vi "Pull Behavior_MWMATHIS.vi"(7 "Water Reward File":path=path "C:/Users/Mackenzie Amoroso/Desktop/REWARD_ente7102015") -> ()   [LabVIEW 2012] (continued)
, "mag"=0.0, "move time"=400.0, "timeout"=1000.0, "watertime"=100.0, "magtime"=25.0, "light"=0.0}, {"home Y2"=3.0, "home X2"=2.8, "home Y1"=2.0, "home X1"=2.4, "home TO"=500.0, "start Y2"=2.7, "start X2"=2.35, "start Y1 "=2.0, "start X1"=2.0, "start TO"=0.0, "end Y2"=2.6, "end X2"=2.2, "end Y1"=2.5, "end X1"=1.8, "end TO"=50.0, "mag"=0.0, "move time"=400.0, "timeout"=1000.0, "watertime"=100.0, "magtime"=25.0, "light"=0.0}, {"home Y2"=3.0, "home X2"=2.8, "home Y1"=2.0, "home X1"=2.4, "home TO"=500.0, "start Y2"=2.7, "start X2"=2.35, "start Y1 "=2.0, "start X1"=2.0, "start TO"=0.0, "end Y2"=2.6, "end X2"=2.2, "end Y1"=2.5, "end X1"=1.8, "end TO"=50.0, "mag"=0.0, "move time"=400.0, "timeout"=1000.0, "watertime"=100.0, "magtime"=25.0, "light"=0.0}, {"home Y2"=3.0, "home X2"=2.8, "home Y1"=2.0, "home X1"=2.4, "home TO"=500.0, "start Y2"=2.7, "start X2"=2.35, "start Y1 "=2.0, "start X1"=2.0, "start TO"=0.0, "end Y2"=2.6, "end X2"=2.2, "end Y1"=2.5, "end X1"=1.8, "end TO"=50.0, "mag"=0.0, "move time"=400.0, "timeout"=1000.0, "watertime"=100.0, "magtime"=25.0, "light"=0.0}, {"home Y2"=3.0, "home X2"=2.8, "home Y1"=2.0, "home X1"=2.4, "home TO"=500.0, "start Y2"=2.7, "start X2"=2.35, "start Y1 "=2.0, "start X1"=2.0, "start TO"=0.0, "end Y2"=2.6, "end X2"=2.2, "end Y1"=2.5, "end X1"=1.8, "end TO"=50.0, "mag"=0.0, "move time"=400.0, "timeout"=1000.0, "watertime"=100.0, "magtime"=25.0, "light"=0.0}, {"home Y2"=3.0, "home X2"=2.8, "home Y1"=2.0, "home X1"=2.4, "home TO"=500.0, "start Y2"=2.7, "start X2"=2.35, "start Y1 "=2.0, "start X1"=2.0, "start TO"=0.0, "end Y2"=2.6, "end X2"=2.2, "end Y1"=2.5, "end X1"=1.8, "end TO"=50.0, "mag"=0.0, "move time"=400.0, "timeout"=1000.0, "watertime"=100.0, "magtime"=25.0, "light"=0.0}, {"home Y2"=3.0, "home X2"=2.8, "home Y1"=2.0, "home X1"=2.4, "home TO"=500.0, "start Y2"=2.7, "start X2"=2.35, "start Y1 "=2.0, "start X1"=2.0, "start TO"=0.0, "end Y2"=2.6, "end X2"=2.2, "end Y1"=2.5, "end X1"=1.8, "end TO"=50.0, "mag"=0.0, "move time"=400.0, "timeout"=1000.0, "watertime"=100.0, "magtime"=25.0, "light"=0.0}, {"home Y2"=3.0, "home X2"=2.8, "home Y1"=2.0, "home X1"=2.4, "home TO"=500.0, "start Y2"=2.7, "start X2"=2.35, "start Y1 "=2.0, "start X1"=2.0, "start TO"=0.0, "end Y2"=2.6, "end X2"=2.2, "end Y1"=2.5, "end X1"=1.8, "end TO"=50.0, "mag"=0.0, "move time"=400.0, "timeout"=1000.0, "watertime"=100.0, "magtime"=25.0, "light"=0.0}, {"home Y2"=3.0, "home X2"=2.8, "home Y1"=2.0, "home X1"=2.4, "home TO"=500.0, "start Y2"=2.7, "start X2"=2.35, "start Y1 "=2.0, "start X1"=2.0, "start TO"=0.0, "end Y2"=2.6, "end X2"=2.2, "end Y1"=2.5, "end X1"=1.8, "end TO"=50.0, "mag"=0.0, "move time"=400.0, "timeout"=1000.0, "watertime"=100.0, "magtime"=25.0, "light"=0.0}, {"home Y2"=3.0, "home X2"=2.8, "home Y1"=2.0, "home X1"=2.4, "home TO"=500.0, "start Y2"=2.7, "start X2"=2.35, "start Y1 "=2.0, "start X1"=2.0, "start TO"=0.0, "end Y2"=2.6, "end X2"=2.2, "end Y1"=2.5, "end X1"=1.8, "end TO"=50.0, "mag"=0.0, "move time"=400.0, "timeout"=1000.0, "watertime"=100.0, "magtime"=25.0, "light"=0.0}, {"home Y2"=3.0, "home X2"=2.8, "home Y1"=2.0, "home X1"=2.4, "home TO"=500.0, "start Y2"=2.7, "start X2"=2.35, "start Y1 "=2.0, "start X1"=2.0, "start TO"=0.0, "end Y2"=2.6, "end X2"=2.2, "end Y1"=2.5, "end X1"=1.8, "end TO"=50.0, "mag"=0.0, "move time"=400.0, "timeout"=1000.0, "watertime"=100.0, "magtime"=25.0, "light"=0.0}, {"home Y2"=3.0, "home X2"=2.8, "home Y1"=2.0, "home X1"=2.4, "home TO"=500.0, "start Y2"=2.7, "start X2"=2.35, "start Y1 "=2.0, "start X1"=2.0, "start TO"=0.0, "end Y2"=2.6, "end X2"=2.2, "end Y1"=2.5, "end X1"=1.8, "end TO"=50.0, "mag"=0.0, "move time"=400.0, "timeout"=1000.0, "watertime"=100.0, "magtime"=25.0, "light"=0.0}, {"home Y2"=3.0, "home X2"=2.8, "home Y1"=2.0, "home X1"=2.4, "home TO"=500.0, "start Y2"=2.7, "start X2"=2.35, "start Y1 "=2.0, "start X1"=2.0, "start TO"=0.0, "end Y2"=2.6, "end X2"=2.2, "end Y1"=2.5, "end X1"=1.8, "end TO"=50.0, "mag"=0.0, "move time"=400.0, "timeout"=1000.0, "watertime"=100.0, "magtime"=25.0, "light"=0.0}, {"home Y2"=3.0, "home X2"=2.8, "home Y1"=2.0, "home X1"=2.4, "home TO"=500.0, "start Y2"=2.7, "start X2"=2.35, "start Y1 "=2.0, "start X1"=2.0, "start TO"=0.0, "end Y2"=2.6, "end X2"=2.2, "end Y1"=2.5, "end X1"=1.8, "end TO"=50.0, "mag"=0.0, "move time"=400.0, "timeout"=1000.0, "watertime"=100.0, "magtime"=25.0, "light"=0.0}, {"home Y2"=3.0, "home X2"=2.8, "home Y1"=2.0, "home X1"=2.4, "home TO"=500.0, "start Y2"=2.7, "start X2"=2.35, "start Y1 "=2.0, "start X1"=2.0, "start TO"=0.0, "end Y2"=2.6, "end X2"=2.2, "end Y1"=2.5, "end X1"=1.8, "end TO"=50.0, "mag"=0.0, "move time"=400.0, "timeout"=1000.0, "watertime"=100.0, "magtime"=25.0, "light"=0.0}, {"home Y2"=3.0, "home X2"=2.8, "home Y1"=2.0, "home X1"=2.4, "home TO"=500.0, "start Y2"=2.7, "start X2"=2.35, "start Y1 "=2.0, "start X1"=2.0, "start TO"=0.0, "end Y2"=2.6, "end X2"=2.2, "end Y1"=2.5, "end X1"=1.8, "end TO"=50.0, "mag"=0.0, "move time"=400.0, "timeout"=1000.0, "watertime"=100.0, "magtime"=25.0, "light"=0.0}, {"home Y2"=3.0, "home X2"=2.8, "home Y1"=2.0, "home X1"=2.4, "home TO"=500.0, "start Y2"=2.7, "start X2"=2.35, "start Y1 "=2.0, "start X1"=2.0, "start TO"=0.0, "end Y2"=2.6, "end X2"=2.2, "end Y1"=2.5, "end X1"=1.8, "end TO"=50.0, "mag"=0.0, "move time"=400.0, "timeout"=1000.0, "watertime"=100.0, "magtime"=25.0, "light"=0.0}, {"home Y2"=3.0, "home X2"=2.8, "home Y1"=2.0, "home X1"=2.4, "home TO"=500.0, "start Y2"=2.7, "start X2"=2.35, "start Y1 "=2.0, "start X1"=2.0, "start TO"=0.0, "end Y2"=2.6, "end X2"=2.2, "end Y1"=2.5, "end X1"=1.8, "end TO"=50.0, "mag"=0.0, "move time"=400.0, "timeout"=1000.0, "watertime"=100.0, "magtime"=25.0, "light"=0.0}, {"home Y2"=3.0, "home X2"=2.8, "home Y1"=2.0, "home X1"=2.4, "home TO"=500.0, "start Y2"=2.7, "start X2"=2.35, "start Y1 "=2.0, "start X1"=2.0, "start TO"=0.0, "end Y2"=2.6, "end X2"=2.2, "end Y1"=2.5, "end X1"=1.8, "end TO"=50.0, "mag"=0.0, "move time"=400.0, "timeout"=1000.0, "watertime"=100.0, "magtime"=25.0, "light"=0.0}, {"home Y2"=3.0, "home X2"=2.8, "home Y1"=2.0, "home X1"=2.4, "home TO"=500.0, "start Y2"=2.7, "start X2"=2.35, "start Y1 "=2.0, "start X1"=2.0, "start TO"=0.0, "end Y2"=2.6, "end X2"=2.2, "end Y1"=2.5, "end X1"=1.8, "end TO"=50.0, "mag"=0.0, "move time"=400.0, "timeout"=1000.0, "watertime"=100.0, "magtime"=25.0, "light"=0.0}, {"home Y2"=3.0, "home X2"=2.8, "home Y1"=2.0, "home X1"=2.4, "home TO"=500.0, "start Y2"=2.7, "start X2"=2.35, "start Y1 "=2.0, "start X1"=2.0, "start TO"=0.0, "end Y2"=2.6, "end X2"=2.2, "end Y1"=2.5, "end X1"=1.8, "end TO"=50.0, "mag"=0.0, "move time"=400.0, "timeout"=1000.0, "watertime"=100.0, "magtime"=25.0, "light"=0.0}, {"home Y2"=3.0, "home X2"=2.8, "home Y1"=2.0, "home X1"=2.4, "home TO"=500.0, "start Y2"=2.7, "start X2"=2.35, "start Y1 "=2.0, "start X1"=2.0, "start TO"=0.0, "end Y2"=2.6, "end X2"=2.2, "end Y1"=2.5, "end X1"=1.8, "end TO"=50.0, "mag"=0.0, "move time"=400.0, "timeout"=1000.0, "watertime"=100.0, "magtime"=25.0, "light"=0.0}, {"home Y2"=3.0, "home X2"=2.8, "home Y1"=2.0, "home X1"=2.4, "home TO"=500.0, "start Y2"=2.7, "start X2"=2.35, "start Y1 "=2.0, "start X1"=2.0, "start TO"=0.0, "end Y2"=2.6, "end X2"=2.2, "end Y1"=2.5, "end X1"=1.8, "end TO"=50.0, "mag"=0.0, "move time"=400.0, "timeout"=1000.0, "watertime"=100.0, "magtime"=25.0, "light"=0.0}, {"home Y2"=3.0, "home X2"=2.8, "home Y1"=2.0, "home X1"=2.4, "home TO"=500.0, "start Y2"=2.7, "start X2"=2.35, "start Y1 "=2.0, "start X1"=2.0, "start TO"=0.0, "end Y2"=2.6, "end X2"=2.2, "end Y1"=2.5, "end X1"=1.8, "end TO"=50.0, "mag"=0.0, "move time"=400.0, "timeout"=1000.0, "watertime"=100.0, "magtime"=25.0, "light"=0.0}, {"home Y2"=3.0, "home X2"=2.8, "home Y1"=2.0, "home X1"=2.4, "home TO"=500.0, "start Y2"=2.7, "start X2"=2.35, "start Y1 "=2.0, "start X1"=2.0, "start TO"=0.0, "end Y2"=2.6, "end X2"=2.2, "end Y1"=2.5, "end X1"=1.8, "end TO"=50.0, "mag"=0.0, "move time"=400.0, "timeout"=1000.0, "watertime"=100.0, "magtime"=25.0, "light"=0.0}, {"home Y2"=3.0, "home X2"=2.8, "home Y1"=2.0, "home X1"=2.4, "home TO"=500.0, "start Y2"=2.7, "start X2"=2.35, "start Y1 "=2.0, "start X1"=2.0, "start TO"=0.0, "end Y2"=2.6, "end X2"=2.2, "end Y1"=2.5, "end X1"=1.8, "end TO"=50.0, "mag"=0.0, "move time"=400.0, "timeout"=1000.0, "watertime"=100.0, "magtime"=25.0, "light"=0.0}, {"home Y2"=3.0, "home X2"=2.8, "home Y1"=2.0, "home X1"=2.4, "home TO"=500.0, "start Y2"=2.7, "start X2"=2.35, "start Y1 "=2.0, "start X1"=2.0, "start TO"=0.0, "end Y2"=2.6, "end X2"=2.2, "end Y1"=2.5, "end X1"=1.8, "end TO"=50.0, "mag"=0.0, "move time"=400.0, "timeout"=1000.0, "watertime"=100.0, "magtime"=25.0, "light"=0.0}, {"home Y2"=3.0, "home X2"=2.8, "home Y1"=2.0, "home X1"=2.4, "home TO"=500.0, "start Y2"=2.7, "start X2"=2.35, "start Y1 "=2.0, "start X1"=2.0, "start TO"=0.0, "end Y2"=2.6, "end X2"=2.2, "end Y1"=2.5, "end X1"=1.8, "end TO"=50.0, "mag"=0.0, "move time"=400.0, "timeout"=1000.0, "watertime"=100.0, "magtime"=25.0, "light"=0.0}, {"home Y2"=3.0, "home X2"=2.8, "home Y1"=2.0, "home X1"=2.4, "home TO"=500.0, "start Y2"=2.7, "start X2"=2.35, "start Y1 "=2.0, "start X1"=2.0, "start TO"=0.0, "end Y2"=2.6, "end X2"=2.2, "end Y1"=2.5, "end X1"=1.8, "end TO"=50.0, "mag"=0.0, "move time"=400.0, "timeout"=1000.0, "watertime"=100.0, "magtime"=25.0, "light"=0.0}, {"home Y2"=3.0, "home X2"=2.8, "home Y1"=2.0, "home X1"=2.4, "home TO"=500.0, "start Y2"=2.7, "start X2"=2.35, "start Y1 "=2.0, "start X1"=2.0, "start TO"=0.0, "end Y2"=2.6, "end X2"=2.2, "end Y1"=2.5, "end X1"=1.8, "end TO"=50.0, "mag"=0.0, "move time"=400.0, "timeout"=1000.0, "watertime"=100.0, "magtime"=25.0, "light"=0.0}, {"home Y2"=3.0, "home X2"=2.8, "home Y1"=2.0, "home X1"=2.4, "home TO"=500.0, "start Y2"=2.7, "start X2"=2.35, "start Y1 "=2.0, "start X1"=2.0, "start TO"=0.0, "end Y2"=2.6, "end X2"=2.2, "end Y1"=2.5, "end X1"=1.8, "end TO"=50.0, "mag"=0.0, "move time"=400.0, "timeout"=1000.0, "watertime"=100.0, "magtime"=25.0, "light"=0.0}, {"home Y2"=3.0, "home X2"=2.8, "home Y1"=2.0, "home X1"=2.4, "home TO"=500.0, "start Y2"=2.7, "start X2"=2.35, "start Y1 "=2.0, "start X1"=2.0, "start TO"=0.0, "end Y2"=2.6, "end X2"=2.2, "end Y1"=2.5, "end X1"=1.8, "end TO"=50.0, "mag"=0.0, "move time"=400.0, "timeout"=1000.0, "watertime"=100.0, "magtime"=25.0, "light"=0.0}, {"home Y2"=3.0, "home X2"=2.8, "home Y1"=2.0, "home X1"=2.4, "home TO"=500.0, "start Y2"=2.7, "start X2"=2.35, "start Y1 "=2.0, "start X1"=2.0, "start TO"=0.0, "end Y2"=2.6, "end X2"=2.2, "end Y1"=2.5, "end X1"=1.8, "end TO"=50.0, "mag"=0.0, "move time"=400.0, "timeout"=1000.0, "watertime"=100.0, "magtime"=25.0, "light"=0.0}, {"home Y2"=3.0, "home X2"=2.8, "home Y1"=2.0, "home X1"=2.4, "home TO"=500.0, "start Y2"=2.7, "start X2"=2.35, "start Y1 "=2.0, "start X1"=2.0, "start TO"=0.0, "end Y2"=2.6, "end X2"=2.2, "end Y1"=2.5, "end X1"=1.8, "end TO"=50.0, "mag"=0.0, "move time"=400.0, "timeout"=1000.0, "watertime"=100.0, "magtime"=25.0, "light"=0.0}, {"home Y2"=3.0, "home X2"=2.8, "home Y1"=2.0, "home X1"=2.4, "home TO"=500.0, "start Y2"=2.7, "start X2"=2.35, "start Y1 "=2.0, "start X1"=2.0, "start TO"=0.0, "end Y2"=2.6, "end X2"=2.2, "end Y1"=2.5, "end X1"=1.8, "end TO"=50.0, "mag"=0.0, "move time"=400.0, "timeout"=1000.0, "watertime"=100.0, "magtime"=25.0, "light"=0.0}, {"home Y2"=3.0, "home X2"=2.8, "home Y1"=2.0, "home X1"=2.4, "home TO"=500.0, "start Y2"=2.7, "start X2"=2.35, "start Y1 "=2.0, "start X1"=2.0, "start TO"=0.0, "end Y2"=2.6, "end X2"=2.2, "end Y1"=2.5, "end X1"=1.8, "end TO"=50.0, "mag"=0.0, "move time"=400.0, "timeout"=1000.0, "watertime"=100.0, "magtime"=25.0, "light"=0.0}, {"home Y2"=3.0, "home X2"=2.8, "home Y1"=2.0, "home X1"=2.4, "home TO"=500.0, "start Y2"=2.7, "start X2"=2.35, "start Y1 "=2.0, "start X1"=2.0, "start TO"=0.0, "end Y2"=2.6, "end X2"=2.2, "end Y1"=2.5, "end X1"=1.8, "end TO"=50.0, "mag"=0.0, "move time"=400.0, "timeout"=1000.0, "watertime"=100.0, "magtime"=25.0, "light"=0.0}, {"home Y2"=3.0, "home X2"=2.8, "home Y1"=2.0, "home X1"=2.4, "home TO"=500.0, "start Y2"=2.7, "start X2"=2.35, "start Y1 "=2.0, "start X1"=2.0, "start TO"=0.0, "end Y2"=2.6, "end X2"=2.2, "end Y1"=2.5, "end X1"=1.8, "end TO"=50.0, "mag"=0.0, "move time"=400.0, "timeout"=1000.0, "watertime"=100.0, "magtime"=25.0, "light"=0.0}, {"home Y2"=0.0, "home X2"=0.0, "home Y1"=0.0, "home X1"=0.0, "home TO"=0.0, "start Y2"=0.0, "start X2"=0.0, "start Y1 "=0.0, "start X1"=0.0, "start TO"=0.0, "end Y2"=0.0, "end X2"=0.0, "end Y1"=0.0, "end X1"=0.0, "end TO"=0.0, "mag"=0.0, "move time"=0.0, "timeout"=0.0, "watertime"=0.0, "magtime"=0.0, "light"=0.0}, {"home Y2"=0.0, "home X2"=0.0, "home Y1"=0.0, "home X1"=0.0, "home TO"=0.0, "start Y2"=0.0, "start X2"=0.0, "start Y1 "=0.0, "start X1"=0.0, "start TO"=0.0, "end Y2"=0.0, "end X2"=0.0, "end Y1"=0.0, "end X1"=0.0, "end TO"=0.0, "mag"=0.0, "move time"=0.0, "timeout"=0.0, "watertime"=0.0, "magtime"=0.0, "light"=0.0}, {"home Y2"=0.0, "home X2"=0.0, "home Y1"=0.0, "home X1"=0.0, "home TO"=0.0, "start Y2"=0.0, "start X2"=0.0, "start Y1 "=0.0, "start X1"=0.0, "start TO"=0.0, "end Y2"=0.0, "end X2"=0.0, "end Y1"=0.0, "end X1"=0.0, "end TO"=0.0, "mag"=0.0, "move time"=0.0, "timeout"=0.0, "watertime"=0.0, "magtime"=0.0, "light"=0.0}, {"home Y2"=0.0, "home X2"=0.0, "home Y1"=0.0, "home X1"=0.0, "home TO"=0.0, "start Y2"=0.0, "start X2"=0.0, "start Y1 "=0.0, "start X1"=0.0, "start TO"=0.0, "end Y2"=0.0, "end X2"=0.0, "end Y1"=0.0, "end X1"=0.0, "end TO"=0.0, "mag"=0.0, "move time"=0.0, "timeout"=0.0, "watertime"=0.0, "magtime"=0.0, "light"=0.0}, {"home Y2"=0.0, "home X2"=0.0, "home Y1"=0.0, "home X1"=0.0, "home TO"=0.0, "start Y2"=0.0, "start X2"=0.0, "start Y1 "=0.0, "start X1"=0.0, "start TO"=0.0, "end Y2"=0.0, "end X2"=0.0, "end Y1"=0.0, "end X1"=0.0, "end TO"=0.0, "mag"=0.0, "move time"=0.0, "timeout"=0.0, "watertime"=0.0, "magtime"=0.0, "light"=0.0}, {"home Y2"=0.0, "home X2"=0.0, "home Y1"=0.0, "home X1"=0.0, "home TO"=0.0, "start Y2"=0.0, "start X2"=0.0, "start Y1 "=0.0, "start X1"=0.0, "start TO"=0.0, "end Y2"=0.0, "end X2"=0.0, "end Y1"=0.0, "end X1"=0.0, "end TO"=0.0, "mag"=0.0, "move time"=0.0, "timeout"=0.0, "watertime"=0.0, "magtime"=0.0, "light"=0.0}, {"home Y2"=0.0, "home X2"=0.0, "home Y1"=0.0, "home X1"=0.0, "home TO"=0.0, "start Y2"=0.0, "start X2"=0.0, "start Y1 "=0.0, "start X1"=0.0, "start TO"=0.0, "end Y2"=0.0, "end X2"=0.0, "end Y1"=0.0, "end X1"=0.0, "end TO"=0.0, "mag"=0.0, "move time"=0.0, "timeout"=0.0, "watertime"=0.0, "magtime"=0.0, "light"=0.0}, {"home Y2"=0.0, "home X2"=0.0, "home Y1"=0.0, "home X1"=0.0, "home TO"=0.0, "start Y2"=0.0, "start X2"=0.0, "start Y1 "=0.0, "start X1"=0.0, "start TO"=0.0, "end Y2"=0.0, "end X2"=0.0, "end Y1"=0.0, "end X1"=0.0, "end TO"=0.0, "mag"=0.0, "move time"=0.0, "timeout"=0.0, "watertime"=0.0, "magtime"=0.0, "light"=0.0}, {"home Y2"=0.0, "home X2"=0.0, "home Y1"=0.0, "home X1"=0.0, "home TO"=0.0, "start Y2"=0.0, "start X2"=0.0, "start Y1 "=0.0, "start X1"=0.0, "start TO"=0.0, "end Y2"=0.0, "end X2"=0.0, "end Y1"=0.0, "end X1"=0.0, "end TO"=0.0, "mag"=0.0, "move time"=0.0, "timeout"=0.0, "watertime"=0.0, "magtime"=0.0, "light"=0.0}, {"home Y2"=0.0, "home X2"=0.0, "home Y1"=0.0, "home X1"=0.0, "home TO"=0.0, "start Y2"=0.0, "start X2"=0.0, "start Y1 "=0.0, "start X1"=0.0, "start TO"=0.0, "end Y2"=0.0, "end X2"=0.0, "end Y1"=0.0, "end X1"=0.0, "end TO"=0.0, "mag"=0.0, "move time"=0.0, "timeout"=0.0, "watertime"=0.0, "magtime"=0.0, "light"=0.0}]
  out "in trigROI":bool
  out "in box begin":u32=1904749424
  in  "exp values":T2
  in  "Load experiment parameters":path=path "C:/Users/Mackenzie Amoroso/Desktop/ExpFiles/experiment paraCT_NEW.05bound_2.2r2.55center.txt"
  out "trial queue":refnum<queue>
  in  "magnet strength (trial)":path=path "C:/Users/Mackenzie Amoroso/Desktop/TRIAL_ente7102015"
  out "queue loop":i32=277971
  out "trail start":u32=1904748688
  in  "Joystick File":path=path "C:/Users/Mackenzie Amoroso/Desktop/joystick_ente7102015"
  out "Trial #":dbl=12.0
  out "start time":u32=1904749089
  out "# elements in queue":i32
  in  "stop":bool
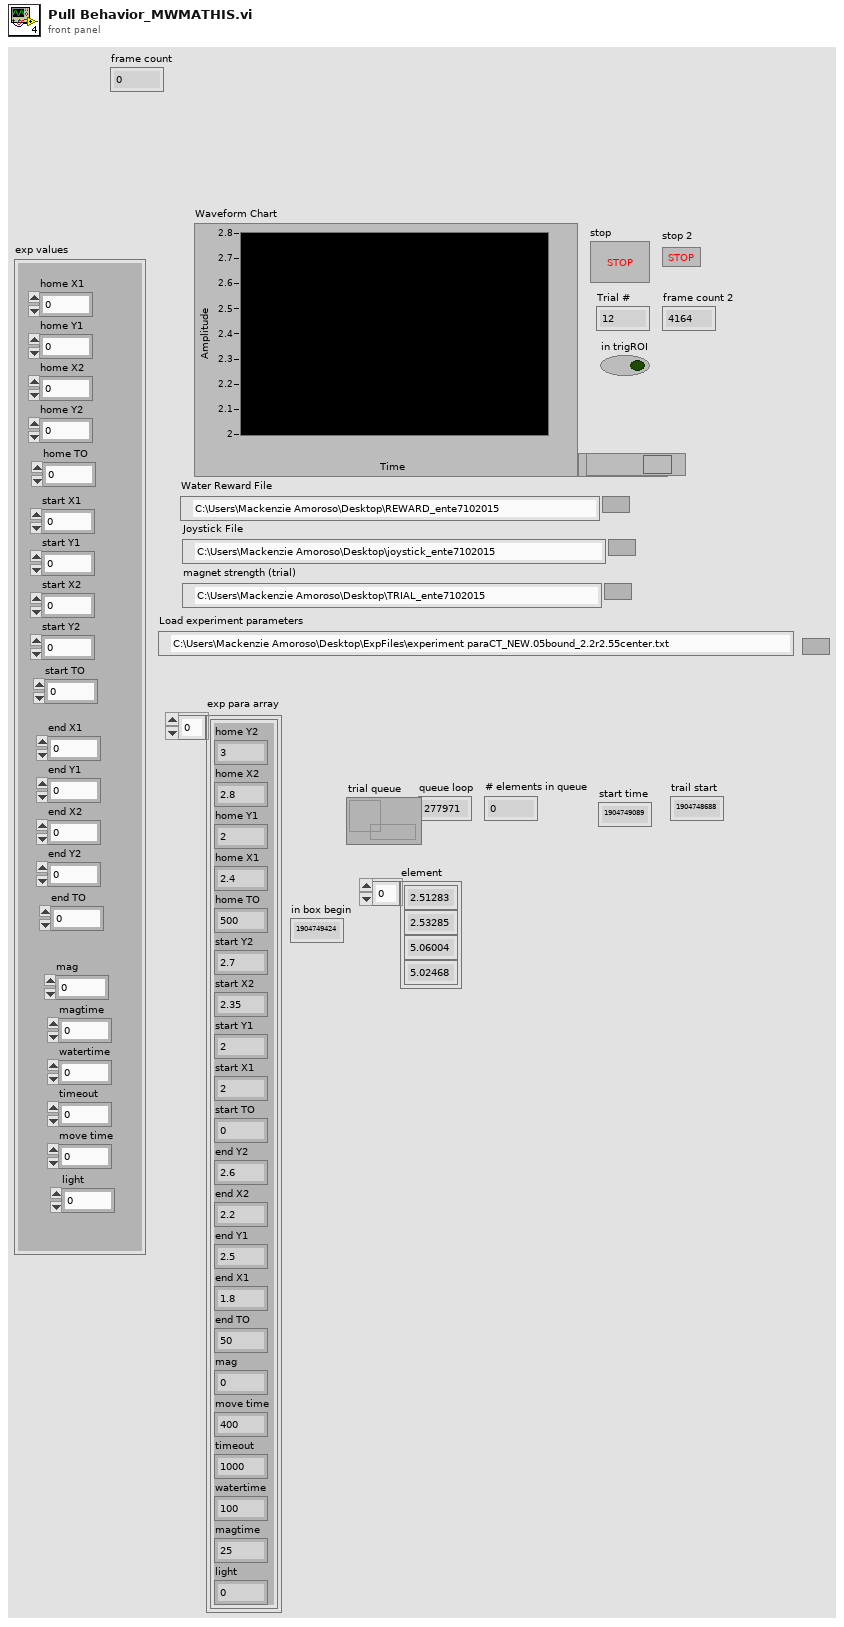
[diagram p1: front panel]
types:
  T1 = cluster{"home Y2":dbl, "home X2":dbl, "home Y1":dbl, "home X1":dbl, "home TO":dbl, "start Y2":dbl, "start X2":dbl, "start Y1 ":dbl, "start X1":dbl, "start TO":dbl, "end Y2":dbl, "end X2":dbl, "end Y1":dbl, "end X1":dbl, "end TO":dbl, "mag":dbl, "move time":dbl, "timeout":dbl, "watertime":dbl, "magtime":dbl, "light":dbl}[]
  T2 = cluster{"home Y2":dbl, "home X2":dbl, "home Y1":dbl, "home X1":dbl, "home TO":dbl, "start Y2":dbl, "start X2":dbl, "start Y1 ":dbl, "start X1":dbl, "start TO":dbl, "end Y2":dbl, "end X2":dbl, "end Y1":dbl, "end X1":dbl, "end TO":dbl, "mag":dbl, "move time":dbl, "timeout":dbl, "watertime":dbl, "magtime":dbl, "light":dbl}
  T3 = enum16{"open", "replace", "create", "open or create", "replace or create", "replace or create with confirmation"}
  T4 = typedef "XDNodeRunTimeDep.lvlib/timing_clust.ctl" = cluster{"Expected End [f-1]":u64, "Actual End [f-1]":u64, "Finished Late? [f-1]":bool, "Expected End [i-1]":u64, "Actual End [i-1]":u64, "Finished Late? [i-1]":bool, "Expected Start [i]":u64, "Actual Start [i]":u64, "Expected Start [f]":u64, "Actual Start [f]":u64, "Source Name":string, "Structure Name":string, "Period":i64, "Deadline":i64, "Offset":i64, "Start":i64, "Priority":i32, "Timeout":i32, "Mode":T5, "Wakeup Reason":T6, "Error":errorcluster, "Source Type":string, "Secondary Source Type":string, "Global End Time":u64, "Global Start Time":u64, "Frame Duration":u64, "Iteration Duration":u64, "Assigned CPU":i32, "I/O Scan Engine Mode":u32}
  T5 = typedef "XDNodeRunTimeDep.lvlib/nitl_modes.ctl" = enum32{"No Change", "Process missed periods, maintain original phase", "Discard missed periods, maintain original phase", "Process missed periods, ignore original phase", "Discard missed periods, ignore original phase"}
  T6 = typedef "XDNodeRunTimeDep.lvlib/wakeup.ctl" = enum32{"Normal", "Aborted", "Asynchronous wakeup", "Timing source error", "Timed loop error", "Timeout"}
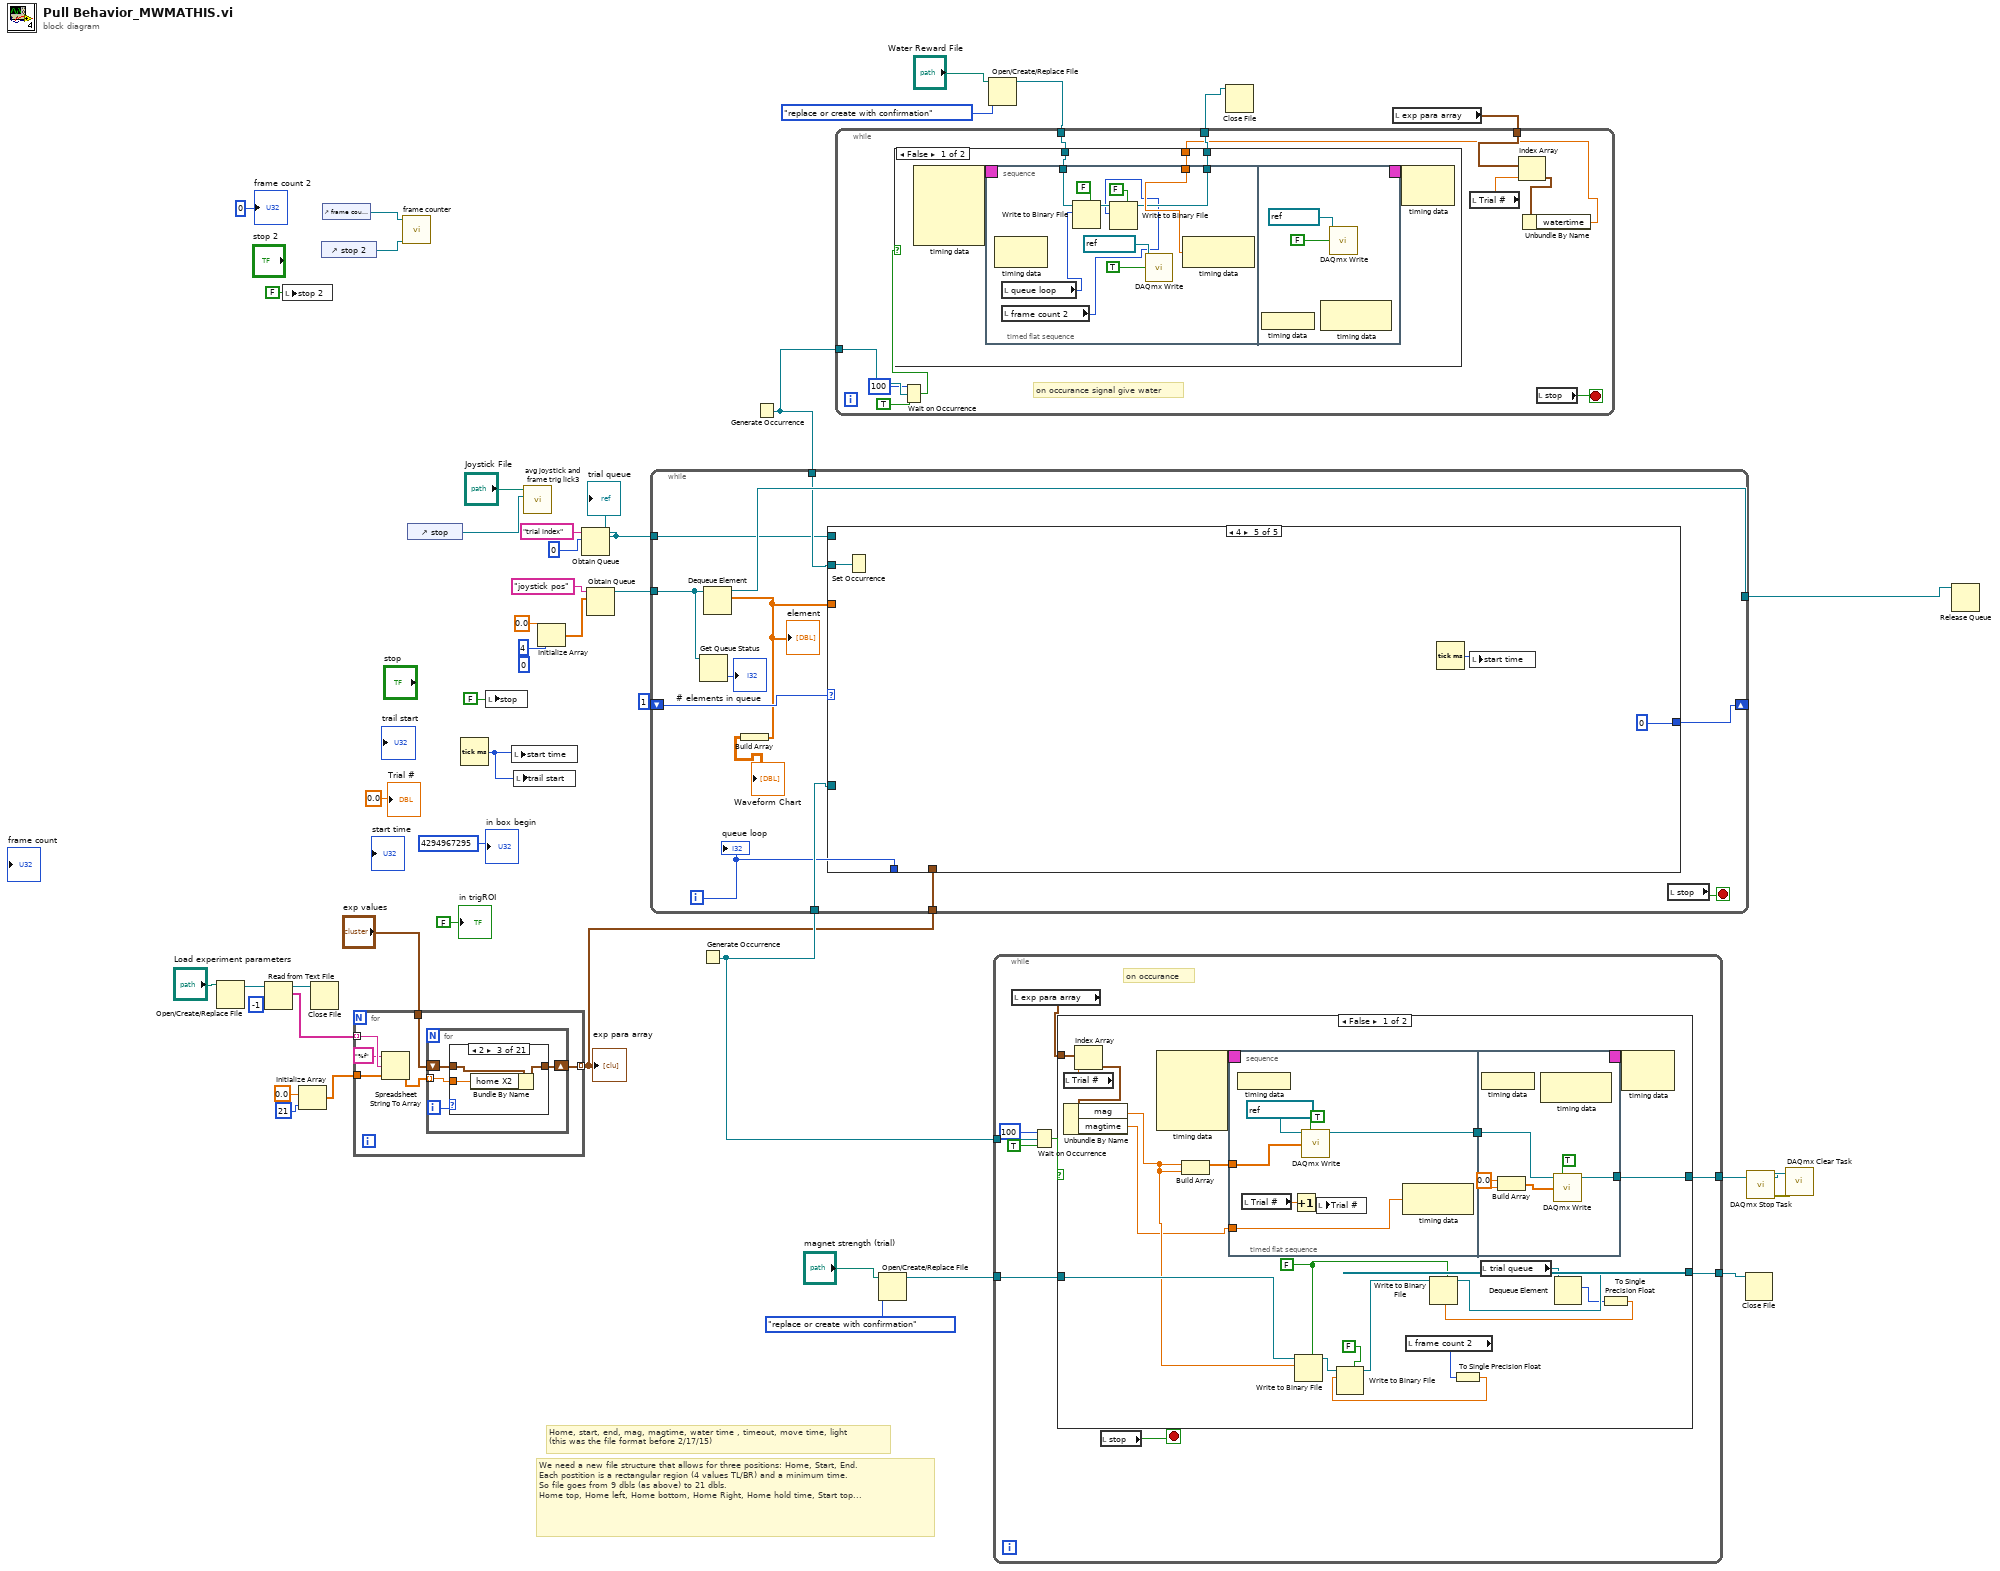
[diagram p0: block diagram]
diagram:
  (unwired) 0 ("dimension size")
  # "We need a new file structure that allows for three positions: Home, Start, End.\nEach postition is a rectangular region (4 values TL/BR) and a minimum time. \nSo file goes from 9 dbls (as above) to 21 dbls. \nHome top, Home left, Home bottom, Home Right, Home hold time, Start top..."
  # "Home, start, end, mag, magtime, water time , timeout, move time, light\n(this was the file format before 2/17/15)"
  n1 = Open/Create/Replace File(file path (use dialog)="Load experiment parameters") -> (refnum out=w16:refnum<file>)  [unwired: 5 in, 2 out]
  n2 = Read from Text File(file (use dialog)=w16, count=-1) -> (refnum out=w13:refnum<file>, text=w14:string[])  [unwired: 2 in, 2 out]
  n3 = local write "stop 2"(FALSE ("stop")) -> ()
  n4 = Initialize Array(0.0 ("element"), 21 ("dimension size")) -> (w10:dbl[])
  n5 = Close File(refnum=w13) -> ()  [unwired: 1 in, 2 out]
  n6 = control-ref of="stop 2"() -> (w3:refnum<vi>)
  n7 = control-ref of="frame count 2"() -> (w4:refnum<vi>)
  n8 = for {
    tunnel: w14 -> [w51] mode=indexing
    tunnel: w10 -> [w49]
    tunnel: "exp values" -> [w47]
    tunnel: [w46] -> w5 mode=indexing
    n9 = Spreadsheet String To Array(format string="%f", spreadsheet string=w51, array type (2D Dbl)=w49) -> (array=w48:dbl[])  [unwired: 1 in]
    n10 = for {
      tunnel: w48 -> [w55] mode=indexing
      shift-right: [w54] -> w46
      shift-left: w47 -> [w53]
      i -> [w52]
      n11 = case shown="2" w52 {
        tunnel: w55 -> [w56 w61 w64 w67 w70 w73 w76 w79 w82 w85 w88 w91 w94 w97 w100 w103 w106 w109 w112 w115 w118]
        tunnel: [w57 w60 w63 w66 w69 w72 w75 w78 w81 w84 w87 w90 w93 w96 w99 w102 w105 w108 w111 w114 w117] -> w54
        tunnel: w53 -> [w58 w59 w62 w65 w68 w71 w74 w77 w80 w83 w86 w89 w92 w95 w98 w101 w104 w107 w110 w113 w116]
        frame 0, Default {
          n12 = Bundle By Name(cluster=w58, "home X1"=w56) -> (w57:T2)
        }
        frame 1 {
          n13 = Bundle By Name(cluster=w59, "home Y1"=w61) -> (w60:T2)
        }
        frame 2 {
          n14 = Bundle By Name(cluster=w62, "home X2"=w64) -> (w63:T2)
        }
        frame 3 {
          n15 = Bundle By Name(cluster=w65, "home Y2"=w67) -> (w66:T2)
        }
        frame 4 {
          n16 = Bundle By Name(cluster=w68, "home TO"=w70) -> (w69:T2)
        }
        frame 5 {
          n17 = Bundle By Name(cluster=w71, "start X1"=w73) -> (w72:T2)
        }
        frame 6 {
          n18 = Bundle By Name(cluster=w74, "start Y1"=w76) -> (w75:T2)
        }
        frame 7 {
          n19 = Bundle By Name(cluster=w77, "start X2"=w79) -> (w78:T2)
        }
        frame 8 {
          n20 = Bundle By Name(cluster=w80, "start Y2"=w82) -> (w81:T2)
        }
        frame 9 {
          n21 = Bundle By Name(cluster=w83, "start TO"=w85) -> (w84:T2)
        }
        frame 10 {
          n22 = Bundle By Name(cluster=w86, "end X1"=w88) -> (w87:T2)
        }
        frame 11 {
          n23 = Bundle By Name(cluster=w89, "end Y1"=w91) -> (w90:T2)
        }
        frame 12 {
          n24 = Bundle By Name(cluster=w92, "end X2"=w94) -> (w93:T2)
        }
        frame 13 {
          n25 = Bundle By Name(cluster=w95, "end Y2"=w97) -> (w96:T2)
        }
        frame 14 {
          n26 = Bundle By Name(cluster=w98, "end TO"=w100) -> (w99:T2)
        }
        frame 15 {
          n27 = Bundle By Name(cluster=w101, "mag"=w103) -> (w102:T2)
        }
        frame 16 {
          n28 = Bundle By Name(cluster=w104, "magtime"=w106) -> (w105:T2)
        }
        frame 17 {
          n29 = Bundle By Name(cluster=w107, "watertime"=w109) -> (w108:T2)
        }
        frame 18 {
          n30 = Bundle By Name(cluster=w110, "timeout"=w112) -> (w111:T2)
        }
        frame 19 {
          n31 = Bundle By Name(cluster=w113, "move time"=w115) -> (w114:T2)
        }
        frame 20 {
          n32 = Bundle By Name(cluster=w116, "light"=w118) -> (w117:T2)
        }
      }
    }
  }
  "exp para array" <- w5
  n33 = call "frame counter.vi"("stop ref"=w3, "frame count ref"=w4) -> ()  [unwired: 10 in]
  n34 = control-ref of="stop"() -> (w33:refnum<vi>)
  n35 = Tick Count (ms)() -> (millisecond timer value=w25:u32)
  n36 = local write "stop"(FALSE ("stop")) -> ()
  n37 = local write "start time"(w25) -> ()
  n38 = local write "trail start"(w25) -> ()
  n39 = call "avg joystick and frame trig lick3.vi"("stop in"=w33, "Joystick File"="Joystick File") -> ()  [unwired: 10 in]
  n40 = Initialize Array(0.0 ("element"), 4 ("dimension size")) -> (w42:dbl[])
  n41 = Obtain Queue(name (unnamed)="trial index", element data type=0 ("dimension size")) -> (queue out=w18:refnum<queue>)  [unwired: 3 in, 2 out]
  "trial queue" <- w18
  n42 = Obtain Queue(name (unnamed)="joystick pos", element data type=w42) -> (queue out=w41:refnum<queue>)  [unwired: 3 in, 2 out]
  n43 = Generate Occurrence() -> (w31:refnum<k4>)
  n44 = Generate Occurrence() -> (w30:refnum<k4>)
  n45 = while {
    tunnel: w41 -> [w130]
    tunnel: [w131] -> w40
    shift-right: [w126] -> _
    shift-left: 1 ("dimension size") -> [w127]
    tunnel: w31 -> [w125]
    tunnel: w30 -> [w124]
    tunnel: w18 -> [w123]
    tunnel: w5 -> [w121]
    i -> [w122]
    stop <- w128 stop-if-true
    n46 = Get Queue Status(queue=w130) -> (# elements in queue=→"# elements in queue":i32)  [unwired: 2 in, 7 out]
    n47 = Dequeue Element(queue=w130) -> (queue out=w131:refnum<queue>, element=w120:dbl[])  [unwired: 2 in, 2 out]
    "element" <- w120
    n48 = Build Array(w120) -> (→"Waveform Chart":dbl[][])
    n49 = case shown="4" w127 {
      tunnel: w120 -> [w156 w195 _ w222 _]
      tunnel: [w153 w194 3 ("dimension size") w221 0 ("dimension size")] -> w126
      tunnel: w125 -> [_ _ w216 _ _]
      tunnel: w124 -> [_ _ _ _ w266]
      tunnel: w123 -> [_ _ w213 _ _]
      tunnel: w122 -> [_ _ w212 _ _]
      tunnel: w121 -> [w152 w191 _ w219 _]
      frame 0, Default {
        # "check if pull status is in home box for minimal amount of time and that trial timeout ha"
        # "check if pull status is home and that trial timout has expired."
        n50 = local read "Trial #"() -> (w151:dbl)
        n51 = Index Array(array=w156, index #1=0 ("index (row)"), index #2=1 ("index (row)")) -> (element #1=w143:dbl, element #2=w140:dbl)
        n52 = local read "start time"() -> (w149:u32)
        n53 = Index Array(array=w152, index=w151) -> (element=w148:T2)
        n54 = Unbundle By Name(w148) -> ("home X2"=w145:dbl, "home X1"=w144:dbl, "home Y2"=w142:dbl, "home Y1"=w141:dbl, "home TO"=w133:dbl)
        n55 = In Range and Coerce(upper limit=w145, x=w143, lower limit=w144) -> (In Range?=w139:bool)  [unwired: 1 out]
        n56 = In Range and Coerce(upper limit=w142, x=w140, lower limit=w141) -> (In Range?=w138:bool)  [unwired: 1 out]
        n57 = Unbundle By Name(w148) -> ("timeout"=w150:dbl)
        n58 = Tick Count (ms)() -> (millisecond timer value=w157:u32)
        n59 = local read "in trigROI"() -> (w136:bool)
        n60 = And(x=w139, y=w138) -> (x .and. y?=w134:bool)
        n61 = Subtract(x=w157, y=w149) -> (x-y=w158:u32)
        n62 = Not(x=w136) -> (.not. x?=w137:bool)
        n63 = And(x=w137, y=w134) -> (x .and. y?=w135:bool)
        n64 = Greater?(x=w158, y=w150) -> (0:w155:bool)
        n65 = case shown="False" w135 {
          tunnel: w134 -> [w161 _]
          tunnel: w133 -> [w160 _]
          tunnel: [w159 FALSE] -> w132
          frame False {
            n66 = case shown="True" w161 {
              tunnel: w160 -> [_ w165]
              tunnel: [FALSE w164] -> w159
              frame False {
                n67 = local write "in trigROI"(FALSE ("in box")) -> ()
              }
              frame True {
                n68 = local read "in box begin"() -> (w167:u32)
                n69 = Tick Count (ms)() -> (millisecond timer value=w166:u32)
                n70 = Subtract(x=w166, y=w167) -> (x-y=w168:u32)
                n71 = Greater?(x=w168, y=w165) -> (0:w164:bool)
              }
            }
          }
          frame True {
            n72 = Tick Count (ms)() -> (millisecond timer value=w170:u32)
            n73 = local write "in trigROI"(TRUE ("in box")) -> ()
            n74 = local write "in box begin"(w170) -> ()
          }
        }
        n75 = And(x=w132, y=w155) -> (x .and. y?=w154:bool)
        n76 = case shown="False" w154 {
          tunnel: [0 ("dimension size") 1 ("dimension size")] -> w153
          frame False {
          }
          frame True {
            n77 = local write "in trigROI"(FALSE ("in box")) -> ()
          }
        }
      }
      frame 1 {
        # "check if magnet/trial start threshold is reached"
        n78 = local read "Trial #"() -> (w192:dbl)
        n79 = Index Array(array=w195, index #1=0 ("index (row)"), index #2=1 ("index (row)")) -> (element #1=w182:dbl, element #2=w181:dbl)
        n80 = Index Array(array=w191, index=w192) -> (element=w193:T2)
        n81 = Unbundle By Name(w193) -> ("start X2"=w190:dbl, "start X1"=w189:dbl, "start Y2"=w188:dbl, "start Y1"=w187:dbl, "start TO"=w177:dbl)
        n82 = In Range and Coerce(upper limit=w190, x=w182, lower limit=w189) -> (In Range?=w184:bool)  [unwired: 1 out]
        n83 = In Range and Coerce(upper limit=w188, x=w181, lower limit=w187) -> (In Range?=w183:bool)  [unwired: 1 out]
        n84 = local read "in trigROI"() -> (w179:bool)
        n85 = And(x=w184, y=w183) -> (x .and. y?=w176:bool)
        n86 = Not(x=w179) -> (.not. x?=w180:bool)
        n87 = And(x=w180, y=w176) -> (x .and. y?=w178:bool)
        n88 = case shown="False" w178 {
          tunnel: w176 -> [w198 _]
          tunnel: w177 -> [w197 _]
          tunnel: [w196 FALSE] -> w175
          frame False {
            n89 = case shown="True" w198 {
              tunnel: w197 -> [_ w202]
              tunnel: [FALSE w201] -> w196
              frame False {
                n90 = local write "in trigROI"(FALSE ("in box")) -> ()
              }
              frame True {
                n91 = local read "in box begin"() -> (w204:u32)
                n92 = Tick Count (ms)() -> (millisecond timer value=w203:u32)
                n93 = Subtract(x=w203, y=w204) -> (x-y=w205:u32)
                n94 = Greater?(x=w205, y=w202) -> (0:w201:bool)
              }
            }
          }
          frame True {
            n95 = Tick Count (ms)() -> (millisecond timer value=w207:u32)
            n96 = local write "in trigROI"(TRUE ("in box")) -> ()
            n97 = local write "in box begin"(w207) -> ()
          }
        }
        n98 = case shown="True" w175 {
          tunnel: [1 ("dimension size") 2 ("dimension size")] -> w194
          frame False {
          }
          frame True {
            n99 = local write "in trigROI"(FALSE ("in box")) -> ()
          }
        }
      }
      frame 2 {
        n100 = Set Occurrence(w216) -> ()
        n101 = Tick Count (ms)() -> (millisecond timer value=w214:u32)
        n102 = Enqueue Element(queue=w213, element=w212) -> ()  [unwired: 2 in, 3 out]
        n103 = local write "trail start"(w214) -> ()
      }
      frame 3 {
        n104 = local read "Trial #"() -> (w220:dbl)
        n105 = local read "trail start"() -> (w224:u32)
        n106 = Index Array(array=w219, index=w220) -> (element=w217:T2)
        n107 = Unbundle By Name(w217) -> ("move time"=w218:dbl)
        n108 = Tick Count (ms)() -> (millisecond timer value=w226:u32)
        n109 = Subtract(x=w226, y=w224) -> (x-y=w225:u32)
        n110 = Greater?(x=w225, y=w218) -> (0:w223:bool)
        n111 = case shown="False" w223 {
          tunnel: w222 -> [w244 _]
          tunnel: [w245 0 ("dimension size")] -> w221
          tunnel: w217 -> [w237 _]
          frame False {
            n112 = Unbundle By Name(w237) -> ("end X2"=w236:dbl, "end X1"=w235:dbl, "end Y2"=w234:dbl, "end Y1"=w233:dbl, "end TO"=w229:dbl)
            n113 = Index Array(array=w244, index #1=0 ("index (row)"), index #2=1 ("index (row)")) -> (element #1=w239:dbl, element #2=w238:dbl)
            n114 = local read "in trigROI"() -> (w231:bool)
            n115 = In Range and Coerce(upper limit=w236, x=w239, lower limit=w235) -> (In Range?=w241:bool)  [unwired: 1 out]
            n116 = In Range and Coerce(upper limit=w234, x=w238, lower limit=w233) -> (In Range?=w240:bool)  [unwired: 1 out]
            n117 = And(x=w241, y=w240) -> (x .and. y?=w227:bool)
            n118 = Not(x=w231) -> (.not. x?=w232:bool)
            n119 = And(x=w232, y=w227) -> (x .and. y?=w230:bool)
            n120 = case shown="False" w230 {
              tunnel: w227 -> [w248 _]
              tunnel: w229 -> [w247 _]
              tunnel: [w246 FALSE] -> w228
              frame False {
                n121 = case shown="True" w248 {
                  tunnel: w247 -> [_ w252]
                  tunnel: [FALSE w251] -> w246
                  frame False {
                    n122 = local write "in trigROI"(FALSE ("in box")) -> ()
                  }
                  frame True {
                    n123 = local read "in box begin"() -> (w254:u32)
                    n124 = Tick Count (ms)() -> (millisecond timer value=w253:u32)
                    n125 = Subtract(x=w253, y=w254) -> (x-y=w255:u32)
                    n126 = Greater?(x=w255, y=w252) -> (0:w251:bool)
                  }
                }
              }
              frame True {
                n127 = Tick Count (ms)() -> (millisecond timer value=w257:u32)
                n128 = local write "in trigROI"(TRUE ("in box")) -> ()
                n129 = local write "in box begin"(w257) -> ()
              }
            }
            n130 = case shown="True" w228 {
              tunnel: [3 ("dimension size") 4 ("dimension size")] -> w245
              frame False {
              }
              frame True {
                n131 = local write "in trigROI"(FALSE ("in box")) -> ()
              }
            }
          }
          frame True {
            n132 = Tick Count (ms)() -> (millisecond timer value=w262:u32)
            n133 = local write "start time"(w262) -> ()
          }
        }
      }
      frame 4 {
        n134 = Set Occurrence(w266) -> ()
        n135 = Tick Count (ms)() -> (millisecond timer value=w264:u32)
        n136 = local write "start time"(w264) -> ()
      }
    }
    n137 = local read "stop"() -> (w128:bool)
    "queue loop" <- w122
  }
  n138 = Open/Create/Replace File(file path (use dialog)="magnet strength (trial)", operation (0:open)=T3."replace or create with confirmation") -> (refnum out=w22:refnum<file>)  [unwired: 4 in, 2 out]
  n139 = Open/Create/Replace File(file path (use dialog)="Water Reward File", operation (0:open)=T3."replace or create with confirmation") -> (refnum out=w27:refnum<file>)  [unwired: 4 in, 2 out]
  n140 = while {
    tunnel: [w274] -> w36
    tunnel: w31 -> [w273]
    tunnel: w22 -> [w269]
    tunnel: [w268] -> w21
    stop <- w275 stop-if-true
    # "on occurance"
    n141 = local read "exp para array"() -> (w267:T1)
    n142 = Wait on Occurrence(1:TRUE ("ignore previous (T)"), 2:w273, 3:100 ("ms timeout (-1)")) -> (0:w272:bool)
    n143 = case shown="False" w272 {
      tunnel: [w293 refnum<k21> "Magnets" ("task/channels in")] -> w274
      tunnel: w269 -> [w292 w320]
      tunnel: [w290 w320] -> w268
      tunnel: w267 -> [w285 _]
      frame False {
        w279 = FALSE ("prepend array or string size? (T)")
        n144 = local read "Trial #"() -> (w286:dbl)
        n145 = Index Array(array=w285, index=w286) -> (element=w284:T2)
        n146 = Unbundle By Name(w284) -> ("mag"=w283:dbl, "magtime"=w282:dbl)
        n147 = node-c288() -> (w295:T4)  [unwired: 4 in]
        n148 = Build Array(w283, w283) -> (w291:dbl[])
        n149 = timed-sequence {
          timing: w295 -> [_]
          timing-out: [_] -> w294
          tunnel: [w299] -> w293
          tunnel: w291 -> [w298]
          tunnel: w282 -> [w296]
          n150 = timed-flat-sequence {
            tunnel: w298 -> [w303]
            tunnel: [w305] -> w297
            tunnel: w296 -> [w302]
            tunnel: w297 -> [w312]
            tunnel: [w311] -> w299
            frame #0 {
              n151 = node-c288() -> ()  [unwired: 1 in]
              n152 = local read "Trial #"() -> (w300:dbl)
              n153 = Increment(x=w300) -> (x+1=w301:dbl)
              n154 = call-poly <vilib>:"DAQmx Write.vi"("task/channels in"=refnum<k21> "Magnets", "auto start"=TRUE, "data"=w303) -> ("task out"=w305:refnum<k21>)  [unwired: 10 in, 2 out]
              n155 = local write "Trial #"(w301) -> ()
              n156 = node-c288(w302) -> ()  [unwired: 1 out]
            }
            frame #1 {
              w314 = 0.0 ("element")
              n157 = node-c288() -> ()  [unwired: 1 in]
              n158 = Build Array(w314, w314) -> (w313:dbl[])
              n159 = node-c288() -> ()  [unwired: 1 in, 1 out]
              n160 = call-poly <vilib>:"DAQmx Write.vi"("task/channels in"=w312, "auto start"=TRUE, "data"=w313) -> ("task out"=w311:refnum<k21>)  [unwired: 10 in, 2 out]
            }
          }
        }
